vi "ProdaNG.ProcessStepParam.Set.vi"(8 "error in (no error)":errorcluster, 10 "ProcessStepParam":T1, 11 "dbHandleIn":i32) -> (0 "error out":errorcluster, 2 "ProcessStepParam out":T1, 3 "dbHandle":i32)   [LabVIEW 2016]
doc: "This function returns a product structure for a product, which is identified by a part and a serial number.\nImportant information: The field 'individual' was taken over from the field 'allgemein' of the legacy data directly. Because of this most products have the value 0 further on and only a few the value 1. \nParameter:\nhandle is an Integer, which is returned by the function Login() at the creation of a new connection.\nwabcoPartId is the Id of the part.\nserialNumber is the serial number of the product for the part above.\nproduct is a pointer on a product structure, which is filled if the returncode is 0. The structure must be defined in the calling program.\n\nReturncodes:\n0 No error\n< 0 ORACLE Error code\n6 (ERROR_INVALID_HANDLE) in case of an invalid handle\n1403 Record does not exist"
uses:
  Controls/ProdaNG.ProcessStepParam.ctl
  Controls/ProdaNG.ProcessStepParamSize.ctl
  prodllNG.dll
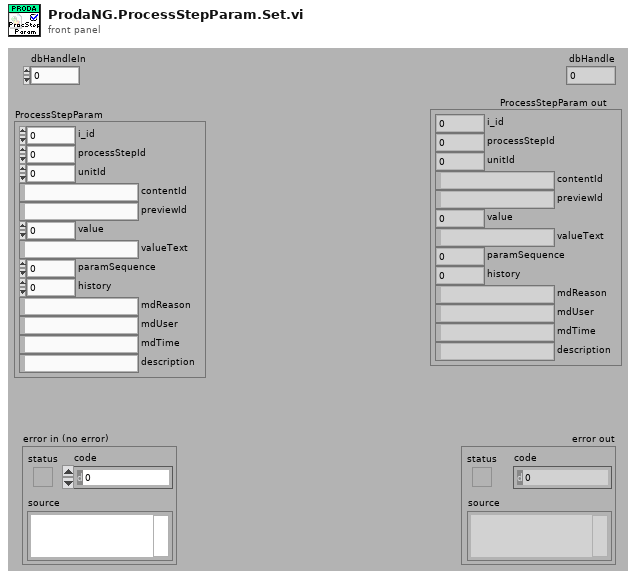
[diagram p1: front panel]
types:
  T1 = typedef "ProdaNG.ProcessStepParam.ctl" = cluster{"i_id":i32, "processStepId":i32, "unitId":i32, "contentId":string, "previewId":string, "value":dbl, "valueText":string, "paramSequence":i32, "history":i32, "mdReason":string, "mdUser":string, "mdTime":string, "description":string}
  T2 = typedef "ProdaNG.ProcessStepParamSize.ctl" = cluster{"i_id":i32, "processStepId":i32, "unitId":i32, "contentId":i32, "previewId":i32, "value":i32, "valueText":i32, "paramSequence":i32, "history":i32, "mdReason":i32, "mdUser":i32, "mdTime":i32, "description":i32}
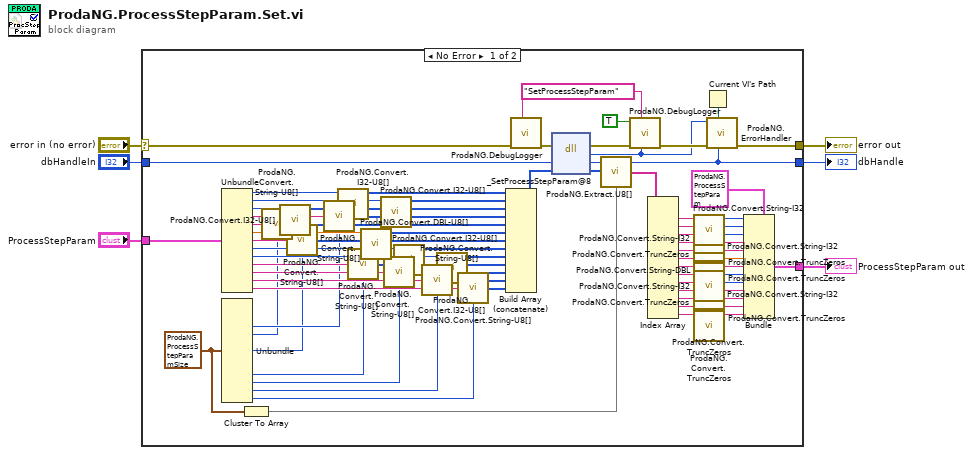
[diagram p0: block diagram]
diagram:
  n1 = case shown="No Error" "error in (no error)" {
    selector: "error in (no error)" -> [w79 w86]
    tunnel: [w84 w86] -> w5
    tunnel: "dbHandleIn" -> [w81 w85]
    tunnel: [w82 w85] -> w3
    tunnel: "ProcessStepParam" -> [w68 _]
    tunnel: [w7 _] -> w1
    frame No Error {
      w69 = T2 {"i_id"=4, "processStepId"=4, "unitId"=4, "contentId"=16, "previewId"=16, "value"=8, "valueText"=258, "paramSequence"=4, "history"=4, "mdReason"=514, "mdUser"=22, "mdTime"=24, "description"=514} ("ProcStepSize")
      w75 = "SetProcessStepParam" ("cmd")
      n2 = Unbundle(w68) -> ("i_id"=w67:i32, "processStepId"=w72:i32, "unitId"=w65:i32, "contentId"=w71:string, "previewId"=w62:string, "value"=w63:dbl, "valueText"=w47:string, "paramSequence"=w45:i32, "history"=w44:i32, "mdReason"=w59:string, "mdUser"=w58:string, "mdTime"=w57:string, "description"=w56:string)
      n3 = Unbundle(w69) -> ("contentId"=w40:i32, "previewId"=w39:i32, "valueText"=w38:i32, "mdReason"=w51:i32, "mdUser"=w50:i32, "mdTime"=w49:i32, "description"=w48:i32)  [unwired: 6 out]
      n4 = Cluster To Array(cluster=w69) -> (array=w36:i32[])
      n5 = call "ProdaNG.Convert.String-U8[].vi"("Input String"=w62, "Size"=w39) -> ("Output"=w61:u8[])
      n6 = call "ProdaNG.Convert.I32-U8[].vi"("32bit integer"=w65) -> ("unsigned byte array"=w64:u8[])  [unwired: 10 in]
      n7 = call "ProdaNG.Convert.String-U8[].vi"("Input String"=w47, "Size"=w38) -> ("Output"=w46:u8[])
      n8 = call "ProdaNG.Convert.String-U8[].vi"("Input String"=w71, "Size"=w40) -> ("Output"=w70:u8[])
      n9 = call "ProdaNG.Convert.I32-U8[].vi"("32bit integer"=w67) -> ("unsigned byte array"=w66:u8[])  [unwired: 10 in]
      n10 = call "ProdaNG.Convert.String-U8[].vi"("Input String"=w59, "Size"=w51) -> ("Output"=w52:u8[])
      n11 = call "ProdaNG.Convert.DBL-U8[].vi"("dbl"=w63) -> ("unsigned byte array"=w60:u8[])  [unwired: 10 in]
      n12 = call "ProdaNG.Convert.I32-U8[].vi"("32bit integer"=w72) -> ("unsigned byte array"=w73:u8[])  [unwired: 10 in]
      n13 = call "ProdaNG.Convert.String-U8[].vi"("Input String"=w58, "Size"=w50) -> ("Output"=w53:u8[])
      n14 = call "ProdaNG.Convert.I32-U8[].vi"("32bit integer"=w45) -> ("unsigned byte array"=w43:u8[])  [unwired: 10 in]
      n15 = call "ProdaNG.Convert.String-U8[].vi"("Input String"=w57, "Size"=w49) -> ("Output"=w54:u8[])
      n16 = call "ProdaNG.Convert.I32-U8[].vi"("32bit integer"=w44) -> ("unsigned byte array"=w42:u8[])  [unwired: 10 in]
      n17 = call "ProdaNG.Convert.String-U8[].vi"("Input String"=w56, "Size"=w48) -> ("Output"=w55:u8[])
      n18 = Build Array (concatenate)(w66, w73, w64, w70, w61, w60, w46, w43, w42, w52, w53, w54, w55) -> (w41:u8[])
      n19 = call "ProdaNG.DebugLogger.vi"("cmd"=w75, "error in (no error)"=w79) -> ("error out"=w78:errorcluster)  [unwired: 9 in]
      n20 = dll-call lib="D:/svn/LineTraceSystem/SOFTWARE/sources/Database/ProdaNG/prodllNG.dll" fn="_SetProcessStepParam@8" ("ProDLL wrapper.dll:ProDLL_wrapper_GetWabcoParts_GetData")(error in=w78, "dbHandle"=w81, "processStepParam"=w41) -> (error out=w77:errorcluster, "return type"=w74:i32, "dbHandle"=w82:i32, "processStepParam"=w37:u8[])  [unwired: 2 in, 1 out]
      n21 = call "ProdaNG.Extract.U8[].vi"("unsigned byte array"=w37, "Sizes"=w36) -> ("Elements"=w35:string[])
      n22 = call "ProdaNG.DebugLogger.vi"("return type"=w74, "cmd"=w75, "error in (no error)"=w77, "done? (F)"=TRUE) -> ("error out"=w76:errorcluster)  [unwired: 7 in]
      n23 = Index Array(array=w35) -> (element #1=w33:string, element #2=w30:string, element #3=w29:string, element #4=w13:string, element #5=w10:string, element #6=w9:string, element #7=w14:string, element #8=w25:string, element #9=w24:string, element #10=w16:string, element #11=w17:string, element #12=w18:string, element #13=w19:string)  [unwired: 13 in]
      n24 = call "ProdaNG.Convert.String-I32.vi"("unsigned byte string"=w33) -> ("32bit integer"=w32:i32)  [unwired: 10 in]
      n25 = call "ProdaNG.Convert.String-I32.vi"("unsigned byte string"=w30) -> ("32bit integer"=w31:i32)  [unwired: 10 in]
      n26 = call "ProdaNG.Convert.String-I32.vi"("unsigned byte string"=w29) -> ("32bit integer"=w28:i32)  [unwired: 10 in]
      n27 = call "ProdaNG.Convert.TruncZeros.vi"("string with \\0s"=w13) -> ("LV string"=w12:string)  [unwired: 10 in]
      n28 = call "ProdaNG.Convert.TruncZeros.vi"("string with \\0s"=w10) -> ("LV string"=w11:string)  [unwired: 10 in]
      n29 = call "ProdaNG.Convert.String-DBL.vi"("unsigned byte string"=w9) -> ("dbl integer"=w8:dbl)  [unwired: 10 in]
      n30 = call "ProdaNG.Convert.TruncZeros.vi"("string with \\0s"=w14) -> ("LV string"=w15:string)  [unwired: 10 in]
      n31 = call "ProdaNG.Convert.String-I32.vi"("unsigned byte string"=w25) -> ("32bit integer"=w27:i32)  [unwired: 10 in]
      n32 = call "ProdaNG.Convert.String-I32.vi"("unsigned byte string"=w24) -> ("32bit integer"=w26:i32)  [unwired: 10 in]
      n33 = call "ProdaNG.Convert.TruncZeros.vi"("string with \\0s"=w16) -> ("LV string"=w22:string)  [unwired: 10 in]
      n34 = call "ProdaNG.Convert.TruncZeros.vi"("string with \\0s"=w17) -> ("LV string"=w23:string)  [unwired: 10 in]
      n35 = call "ProdaNG.Convert.TruncZeros.vi"("string with \\0s"=w18) -> ("LV string"=w21:string)  [unwired: 10 in]
      n36 = call "ProdaNG.Convert.TruncZeros.vi"("string with \\0s"=w19) -> ("LV string"=w20:string)  [unwired: 10 in]
      n37 = Current VI's Path() -> (path=w83:path)
      n38 = call "ProdaNG.ErrorHandler.vi"("dbHandleIn"=w82, "Path"=w83, "error in"=w76, "output_parameter"=w74) -> ("error out"=w84:errorcluster)  [unwired: 7 in]
      n39 = Bundle(cluster=T1 {"i_id"=0, "processStepId"=0, "unitId"=0, "contentId"="", "previewId"="", "value"=0.0, "valueText"="", "paramSequence"=0, "history"=0, "mdReason"="", "mdUser"="", "mdTime"="", "description"=""} ("ProcessStepParam"), "i_id"=w32, "processStepId"=w31, "unitId"=w28, "contentId"=w12, "previewId"=w11, "value"=w8, "valueText"=w15, "paramSequence"=w27, "history"=w26, "mdReason"=w22, "mdUser"=w23, "mdTime"=w21, "description"=w20) -> (w7:T1)
    }
    frame Error {
    }
  }
  "error out" <- w5
  "dbHandle" <- w3
  "ProcessStepParam out" <- w1
